vi "Instr_SetPrivateData.vi"(8 "error in (no error)":errorcluster, 11 "LCRControl in":refnum<class "LCRControl.lvclass">) -> (0 "error out":errorcluster, 3 "LCRControl out":refnum<class "LCRControl.lvclass">)   [LabVIEW 2013, in "LCRControl.lvclass"]
uses:
  LCRControl.lvclass
  InstrControl.lvclass
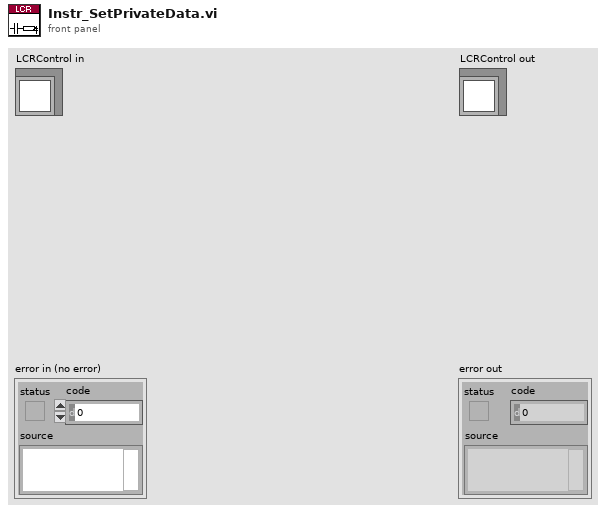
[diagram p1: front panel]
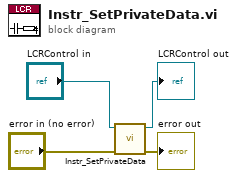
[diagram p0: block diagram]
diagram:
  n1 = call-parent "Instr_SetPrivateData.vi"("error in (no error)"="error in (no error)", "InstrControl in"="LCRControl in") -> ("error out"=→"error out":errorcluster, "InstrControl out"=→"LCRControl out":refnum<class "LCRControl.lvclass">)  [unwired: 8 in]
